vi "Compute DistanceTo Coral Ver 2.vi"(6 "Robot Calibration Cluster":T1={"Camera Height on robot (in)"=6.0, "Camera Angle on the robot (deg)"=5.0, "Camera FOV Top to Bottom View Angle (deg)"=1.0, "Target size (in)"=0.0, "Distance to front of bumper (in)"=9.75} {"Distance to front of bumper (in)" format="%#_13g"; "Target size (in)" format="%#_13g"; "Camera FOV Top to Bottom View Angle (deg)" format="%#_13g"; "Camera Angle on the robot (deg)" format="%#_13g"; "Camera Height on robot (in)" format="%#_13g"}, 9 "Screen resolution pixels Height (Ry)":dbl=600.0 format="%#_13g", 10 "Target Vertical pixels bottom - top (pixels)":dbl=-46.076202392578125 format="%#_13g") -> (3 "Distance from target (in)":dbl format="%.2f")   [LabVIEW 2023]
uses:
  April Tags/Camera Info.ctl
panel:
  # "These Items are inputs"
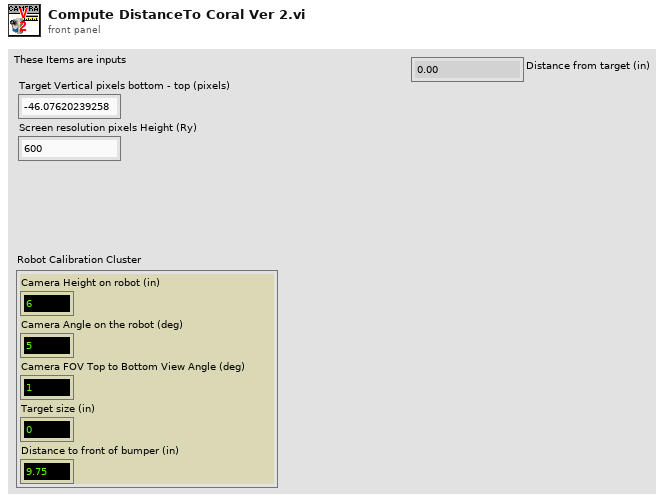
[diagram p1: front panel]
types:
  T1 = typedef "Camera Info.ctl" = cluster{"Camera Height on robot (in)":dbl, "Camera Angle on the robot (deg)":dbl, "Camera FOV Top to Bottom View Angle (deg)":dbl, "Target size (in)":dbl, "Distance to front of bumper (in)":dbl}
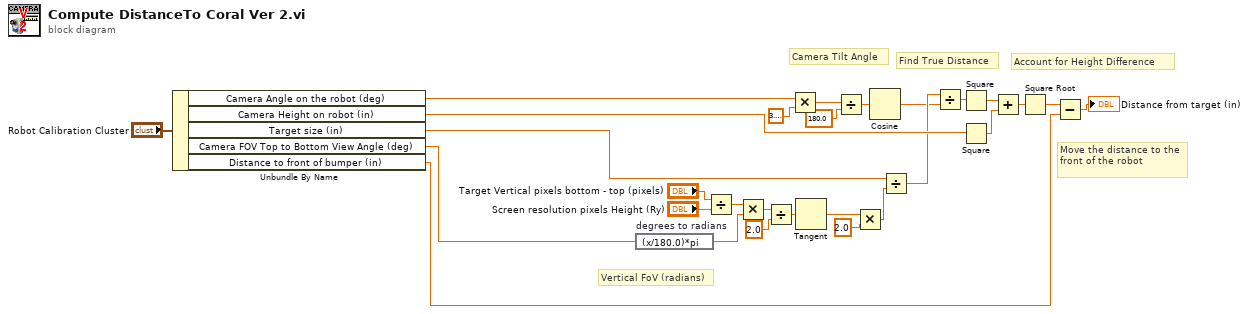
[diagram p0: block diagram]
diagram:
  # "Move the distance to the front of the robot"
  # "Camera Tilt Angle"
  # "Account for Height Difference"
  # "Find True Distance"
  # "Vertical FoV (radians)"
  n1 = Unbundle By Name("Robot Calibration Cluster") -> ("Camera Angle on the robot (deg)"=w13:dbl, "Camera Height on robot (in)"=w25:dbl, "Target size (in)"=w5:dbl, "Camera FOV Top to Bottom View Angle (deg)"=w4:dbl, "Distance to front of bumper (in)"=w1:dbl)
  n2 = expression code="(x/180.0)*pi" "degrees to radians"(w4) -> (w19:dbl)
  n3 = Divide(x="Target Vertical pixels bottom - top (pixels)", y="Screen resolution pixels Height (Ry)") -> (x/y=w20:dbl)
  n4 = Multiply(x=w20, y=w19) -> (x*y=w18:dbl)
  n5 = Divide(x=w18, y=2.0) -> (x/y=w16:dbl)
  n6 = Multiply(x=w13, y=3.141592653589793) -> (x*y=w12:dbl)
  n7 = Tangent(1:w16) -> (0:w15:dbl)
  n8 = Divide(x=w12, y=180.0) -> (x/y=w10:dbl)
  n9 = Multiply(x=w15, y=2.0) -> (x*y=w27:dbl)
  n10 = Cosine(x=w10) -> (cos(x)=w8:dbl)
  n11 = Divide(x=w5, y=w27) -> (x/y=w9:dbl)
  n12 = Divide(x=w9, y=w8) -> (x/y=w7:dbl)
  n13 = Square(x=w7) -> (x^2=w24:dbl)
  n14 = Square(x=w25) -> (x^2=w23:dbl)
  n15 = Add(x=w24, y=w23) -> (x+y=w22:dbl)
  n16 = Square Root(x=w22) -> (sqrt(x)=w2:dbl)
  n17 = Subtract(x=w2, y=w1) -> (x-y=→"Distance from target (in)":dbl)
